vi "vhf_get_iterations.vi"(0 "Right":bool, 1 "Left":bool, 2 "Iterations (Exploded)":dbl, 3 "Start Slice (360/alpha)":dbl, 4 "Number of Bins (360/ VHF resolution)":dbl) -> (5 "Start Slice":dbl, 6 "Number of Iterations":dbl)   [LabVIEW 2010]
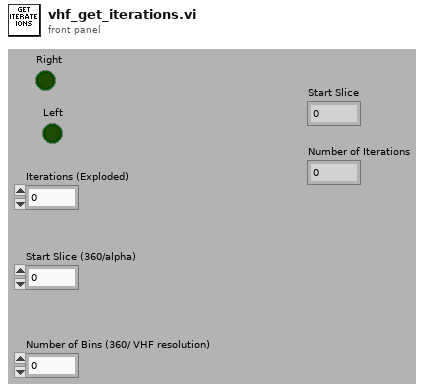
[diagram p1: front panel]
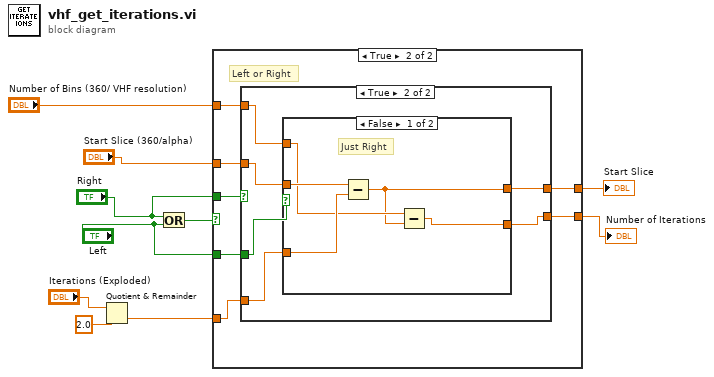
[diagram p0: block diagram]
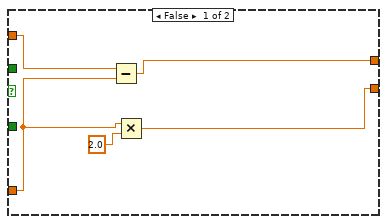
[diagram p2: hidden frame]
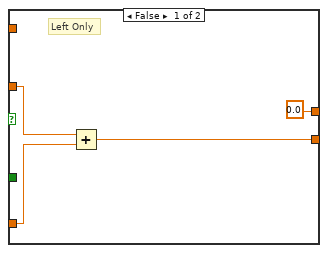
[diagram p3: hidden frame]
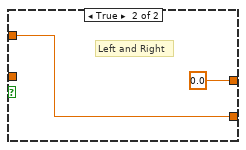
[diagram p4: hidden frame]
diagram:
  n1 = Quotient & Remainder(x="Iterations (Exploded)", y=2.0) -> (floor(x/y)=w5:dbl)  [unwired: 1 out]
  n2 = Or(x="Right", y="Left") -> (x .or. y?=w10:bool)
  n3 = case shown="True" w10 {
    tunnel: "Right" -> [_ w22]
    tunnel: "Left" -> [_ w16]
    tunnel: w5 -> [w13 w18]
    tunnel: [w14 w21] -> w4
    tunnel: "Start Slice (360/alpha)" -> [w15 w20]
    tunnel: "Number of Bins (360/ VHF resolution)" -> [_ w19]
    tunnel: [w11 w17] -> w1
    frame False {
      n4 = Subtract(x=w15, y=w13) -> (x-y=w14:dbl)
      n5 = Multiply(x=w13, y=2.0) -> (x*y=w11:dbl)
    }
    frame True {
      # "Left or Right"
      n6 = case shown="True" w22 {
        tunnel: [0.0 ("y") w29] -> w21
        tunnel: w20 -> [w25 w28]
        tunnel: w19 -> [_ w31]
        tunnel: w18 -> [w24 w27]
        tunnel: [w23 w30] -> w17
        tunnel: w16 -> [_ w32]
        frame False {
          # "Left Only"
          n7 = Add(x=w25, y=w24) -> (x+y=w23:dbl)
        }
        frame True {
          n8 = case shown="False" w32 {
            tunnel: w31 -> [w35 w39]
            tunnel: [w33 w39] -> w30
            tunnel: [w34 0.0 ("y")] -> w29
            tunnel: w28 -> [w37 _]
            tunnel: w27 -> [w36 _]
            frame False {
              # "Just Right"
              n9 = Subtract(x=w37, y=w36) -> (x-y=w34:dbl)
              n10 = Subtract(x=w35, y=w34) -> (x-y=w33:dbl)
            }
            frame True {
              # "Left and Right"
            }
          }
        }
      }
    }
  }
  "Start Slice" <- w4
  "Number of Iterations" <- w1
